vi "DataSockets Write.vi"(8 "Data":variant[](array[variant]), 9 "mode":T1(ring), 10 "Array":string[](array[string]), 11 "Main Path":string) -> (0 "Array Out":errorcluster[](array[cluster]))   [LabVIEW 2014]
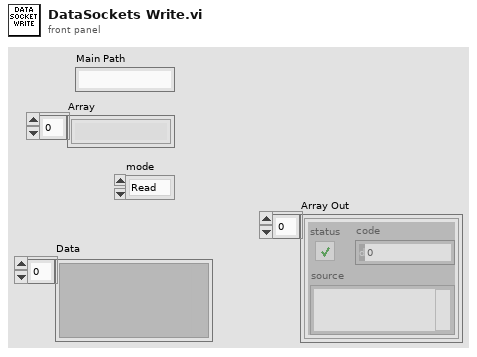
[diagram p1: front panel]
types:
  T1 = enum16{"Read", "Write", "ReadWrite", "BufferedRead", "BufferedReadWrite"}
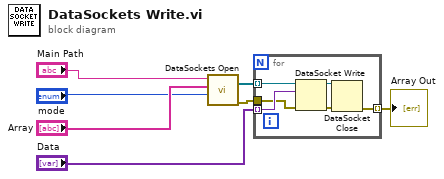
[diagram p0: block diagram]
diagram:
  n1 = call "DataSockets Open.vi"("mode"="mode", "Variables"="Array", "Main Path"="Main Path") -> ("error out"=w1:errorcluster, "Array"=w5:refnum<k13>[])  [unwired: 7 in]
  n2 = for {
    tunnel: w5 -> [w13] mode=indexing
    tunnel: [w10] -> w3 mode=indexing
    tunnel: "Data" -> [w9] mode=indexing
    tunnel: w1 -> [w8]
    n3 = DataSocket Write(8:w8, 10:w9, 11:w13) -> (0:w11:errorcluster, 3:w12:refnum<k13>)  [unwired: 1 in, 1 out]
    n4 = DataSocket Close(8:w11, 11:w12) -> (0:w10:errorcluster)  [unwired: 1 in, 1 out]
  }
  "Array Out" <- w3
